vi "ADCHEXarrTomV.vi"(11 "数组":i32[](array[numeric]), 12 "索引":i32) -> (0 "ADC值":string, 4 "电压mV":dbl, 14 "NEXT":i32)   [LabVIEW 2020]
panel:
  out "ADC值":u32
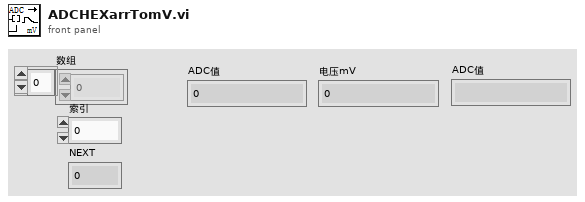
[diagram p1: front panel]
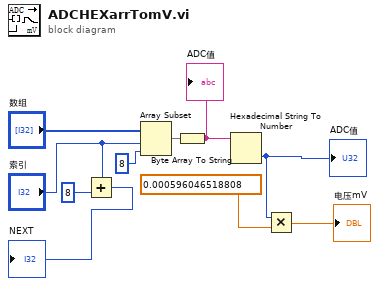
[diagram p0: block diagram]
diagram:
  n1 = Add(x="索引", y=8) -> (x+y=→"NEXT":i32)
  n2 = Array Subset(array="数组", index="索引", length=8 ("长度")) -> (w9:i32[])
  n3 = Byte Array To String(unsigned byte array=w9) -> (string=w8:string)
  "ADC值" <- w8
  n4 = Hexadecimal String To Number(string=w8) -> (number=w6:u32)  [unwired: 2 in, 1 out]
  "ADC值" <- w6
  n5 = Multiply(x=w6, y=0.000596046518808) -> (x*y=→"电压mV":dbl)
